vi "CLC_JIO_Channel.vi"(7 "Channel_setting":T1, 8 "error in":errorcluster) -> (0 "error out":errorcluster, 3 "standard output":string)   [LabVIEW 2023, in "CLC_JIO_FTDI.lvlib"]
uses:
  CLC_JIO_FTDI.lvlib
panel:
  out "standard error":string
  out "floder?":bool
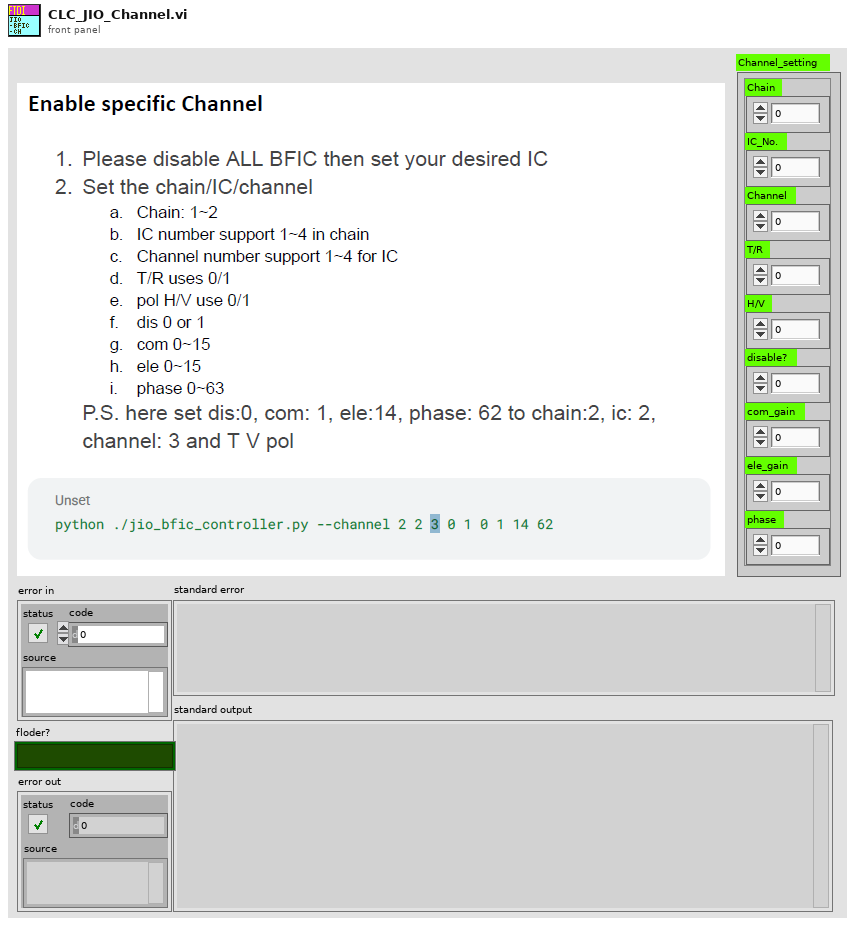
[diagram p1: front panel]
types:
  T1 = cluster{"Chain":i32, "IC_No.":i32, "Channel":i32, "T/R":i32, "H/V":i32, "disable?":i32, "com_gain":i32, "ele_gain":i32, "phase":i32}
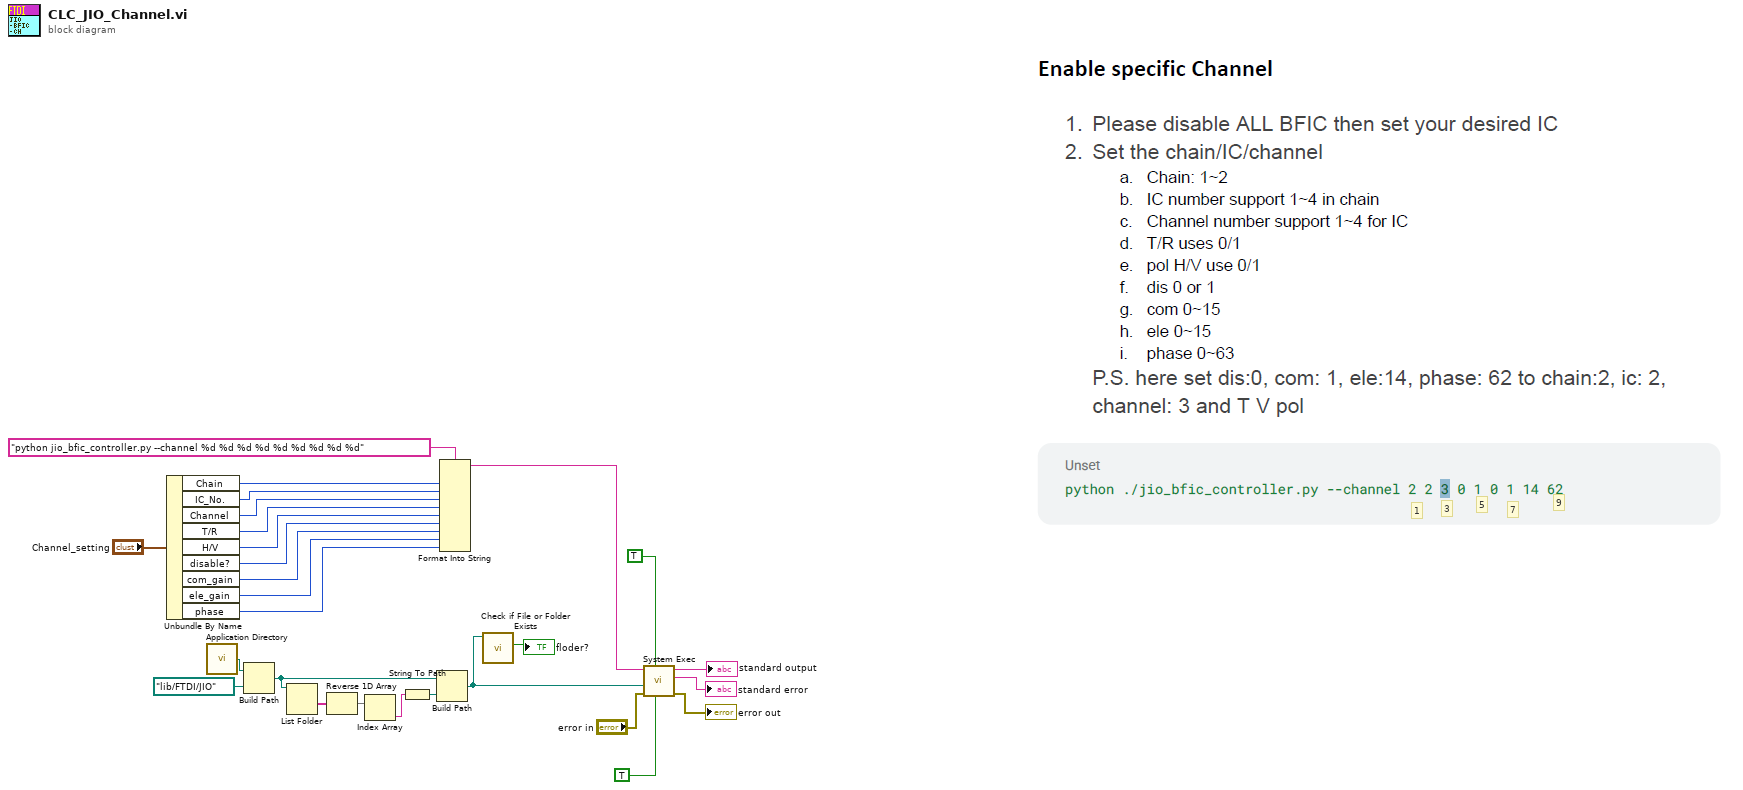
[diagram p0: block diagram]
diagram:
  # "9"
  # "7"
  # "5"
  # "3"
  # "1"
  n1 = Unbundle By Name("Channel_setting") -> ("Chain"=w9:i32, "IC_No."=w8:i32, "Channel"=w7:i32, "T/R"=w6:i32, "H/V"=w5:i32, "disable?"=w4:i32, "com_gain"=w3:i32, "ele_gain"=w2:i32, "phase"=w1:i32)
  n2 = call <vilib>:"Application Directory.vi"() -> ("Application Directory"=w21:path)
  n3 = Build Path(base path=w21, name or relative path=path "lib/FTDI/JIO") -> (appended path=w20:path)
  n4 = List Folder(path=w20) -> (folder names=w26:string[])  [unwired: 3 in, 3 out]
  n5 = Reverse 1D Array(array=w26) -> (reversed array=w25:string[])
  n6 = Index Array(array=w25) -> (element=w24:string)  [unwired: 1 in]
  n7 = String To Path(string=w24) -> (path=w23:path)
  n8 = Build Path(base path=w20, name or relative path=w23) -> (appended path=w18:path)
  n9 = Format Into String(format string="python jio_bfic_controller.py --channel %d %d %d %d %d %d %d %d %d", w9, w8, w7, w6, w5, w4, w3, w2, w1) -> (resulting string=w11:string)  [unwired: 2 in, 1 out]
  n10 = call <vilib>:"Check if File or Folder Exists.vi"("path"=w18) -> ("file or folder exists?"=→"floder?":bool)  [unwired: 8 in, 2 out]
  n11 = call <vilib>:"System Exec.vi"("run minimized? (F)"=TRUE, "wait until completion? (T)"=TRUE, "error in (no error)"="error in", "working directory"=w18, "command line"=w11) -> ("error out"=→"error out":errorcluster, "standard error"=→"standard error":string, "standard output"=→"standard output":string)  [unwired: 3 in, 1 out]
